vi "sequencerGlobVarsWrite.vi"(0 "fpgaState":T1, 2 "cmdByHost":T1, 3 "abort":bool, 4 "halt":bool, 5 "hostConfirmsHzOffsetIsSet":bool) -> ()   [LabVIEW 2014]
uses:
  sequencerState.ctl
  <vilib>/rvi/Emulation/niFpgaSctlEmulationGetInTimedLoop.vi
  sequencerGlobVars.vi
  <vilib>/rvi/Emulation/niFpgaProcessEmulError.vi
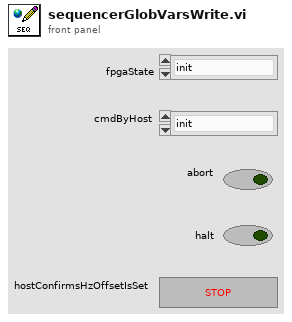
[diagram p1: front panel]
types:
  T1 = typedef "sequencerState.ctl" = enum16{"init", "idle", "writeGlobVars", "measureOffset", "measureTrack", "measComplete", "error"}
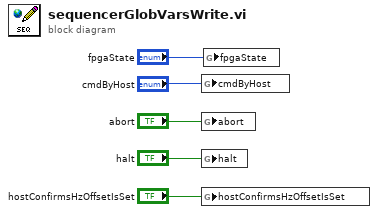
[diagram p0: block diagram]
diagram:
  n1 = global write "sequencerGlobVars.vi" "cmdByHost"("cmdByHost") -> ()
  n2 = global write "sequencerGlobVars.vi" "abort"("abort") -> ()
  n3 = global write "sequencerGlobVars.vi" "halt"("halt") -> ()
  n4 = global write "sequencerGlobVars.vi" "hostConfirmsHzOffsetIsSet"("hostConfirmsHzOffsetIsSet") -> ()
  n5 = global write "sequencerGlobVars.vi" "fpgaState"("fpgaState") -> ()
